vi "parseCommand.vi"(8 "error in (no error)":errorcluster, 11 "MonoCommunicator in":refnum<class "MonoCommunicator.lvclass">) -> (0 "error out":errorcluster, 3 "MonoCommunicator out":refnum<class "MonoCommunicator.lvclass">)   [LabVIEW 2016, in "MonoCommunicator.lvclass"]
uses:
  MonoCommunicator.lvclass
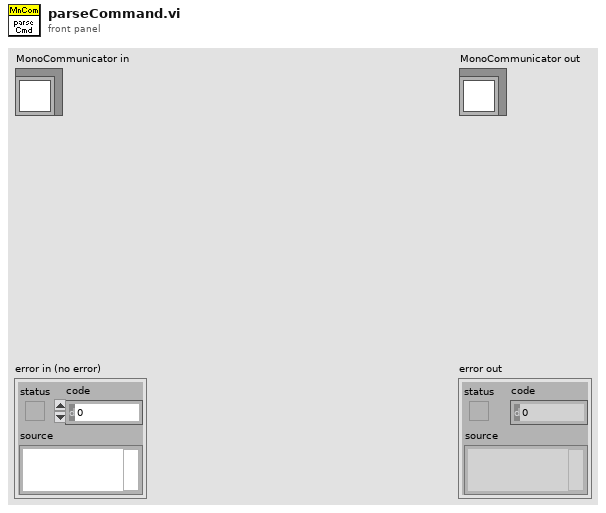
[diagram p1: front panel]
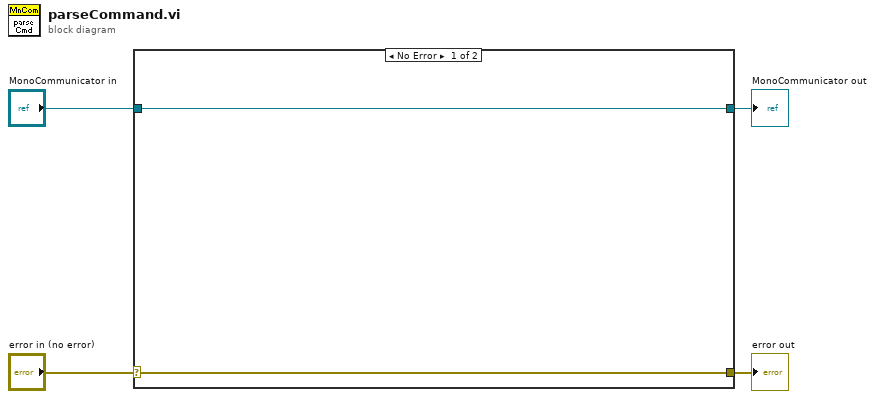
[diagram p0: block diagram]
diagram:
  n1 = case shown="No Error" "error in (no error)" {
    selector: "error in (no error)" -> [w5 w8]
    tunnel: [w5 w8] -> w3
    tunnel: [w6 w7] -> w1
    tunnel: "MonoCommunicator in" -> [w6 w7]
    frame No Error {
    }
    frame Error {
    }
  }
  "error out" <- w3
  "MonoCommunicator out" <- w1
